vi "OpenAllPods.vi"(11 "Configuration Data":T1) -> (3 "All Pods":T18(array[cluster]))   [LabVIEW 2014]
uses:
  <vilib>/Rock Robotics/WPI/MotorControl/WPI_MotorControlDeviceRef.ctl
  <vilib>/Rock Robotics/WPI/MotorControl/WPI_MotorControlType.ctl
  <vilib>/Rock Robotics/SystemInterfaces/Typedef/FPGA_TypedefDigitalModule.ctl
  <vilib>/Rock Robotics/SystemInterfaces/DIO/FPGA_DIOPWMChannel.ctl
  <vilib>/Rock Robotics/WPI/PWM/WPI_PWMDeadband.ctl
  <vilib>/Rock Robotics/WPI/CAN/Jaguar/SubVIs/WPI_CANJaguar_ControlMode.ctl
  <vilib>/Rock Robotics/WPI/CAN/TalonSRX/WPI_CANTalonSRX_APIControlMode.ctl
  <vilib>/Rock Robotics/WPI/PWM/WPI_PWMTransform_ConPane.ctl
  <vilib>/Rock Robotics/WPI/AnalogChannel/WPI_AnalogChannelDevRef.ctl
  <vilib>/Rock Robotics/SystemInterfaces/Typedef/FPGA_TypedefAnalogModule.ctl
  <vilib>/Rock Robotics/SystemInterfaces/AI/FPGA_AIChannel.ctl
  <vilib>/Rock Robotics/WPI/Encoder/WPI_EncoderDevRef.ctl
  <vilib>/Rock Robotics/SystemInterfaces/Encoder/FPGA_EncoderIdx.ctl
  <vilib>/Rock Robotics/SystemInterfaces/Counter/FPGA_CounterCtrSystemIndex.ctl
  <vilib>/Rock Robotics/WPI/Encoder/WPI_EncoderType.ctl
  <vilib>/Rock Robotics/WPI/MotorControl/WPI_MotorControlOpen Talon.vi
  <vilib>/Rock Robotics/WPI/MotorControl/WPI_MotorControlOpenCANTalonSRX.vi
  <vilib>/Rock Robotics/WPI/Counter/WPI_CounterDigitalInputToDigitalSource.vi
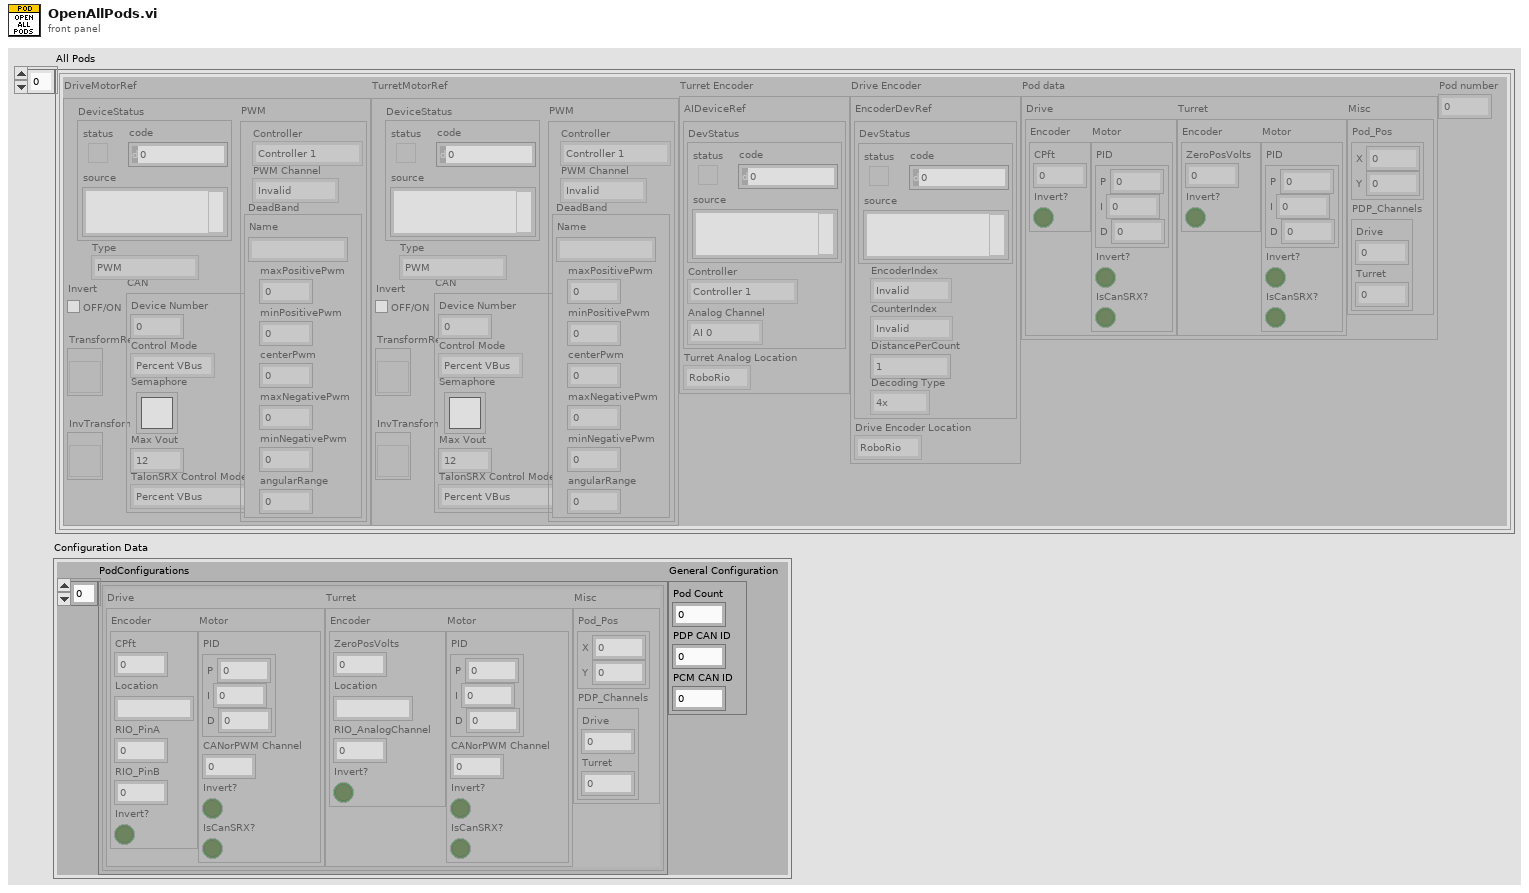
[diagram p1: front panel]
types:
  T1 = cluster{"PodConfigurations":cluster{"Drive":cluster{"Encoder":cluster{"CPft":dbl, "Location":string, "RIO_PinA":i32, "RIO_PinB":i32, "Invert?":bool}, "Motor":cluster{"PID":cluster{"P":dbl, "I":dbl, "D":dbl}, "CANorPWM Channel":i32, "Invert?":bool, "IsCanSRX?":bool}}, "Turret":cluster{"Encoder":cluster{"ZeroPosVolts":dbl, "Location":string, "RIO_AnalogChannel":i32, "Invert?":bool}, "Motor":cluster{"PID":cluster{"P":dbl, "I":dbl, "D":dbl}, "CANorPWM Channel":i32, "Invert?":bool, "IsCanSRX?":bool}}, "Misc":cluster{"Pod_Pos":cluster{"X":dbl, "Y":dbl}, "PDP_Channels":cluster{"Drive":i32, "Turret":i32}}}[], "General Configuration":cluster{"Pod Count":i32, "PDP CAN ID":i32, "PCM CAN ID":i32}}
  T2 = typedef "WPI_MotorControlDeviceRef.ctl" = cluster{"DeviceStatus":errorcluster, "Type":T3, "PWM":cluster{"Controller":T4, "PWM Channel":T5, "DeadBand":T6}, "CAN":cluster{"Device Number":u8, "Control Mode":T7, "Semaphore":T8, "Max Vout":dbl, "TalonSRX Control Mode":T9}, "Invert":bool, "TransformRef":T10, "InvTransformRef":T10}
  T3 = typedef "WPI_MotorControlType.ctl" = enum16{"PWM", "CAN", "CANTalonSRX"}
  T4 = typedef "FPGA_TypedefDigitalModule.ctl" = enum16{"Controller 1"}
  T5 = typedef "FPGA_DIOPWMChannel.ctl" = enum8{"PWM 0", "PWM 1", "PWM 2", "PWM 3", "PWM 4", "PWM 5", "PWM 6", "PWM 7", "PWM 8", "PWM 9", "PWM MXP 0", "PWM MXP 1", "PWM MXP 2", "PWM MXP 3", "PWM MXP 4", "PWM MXP 5", "PWM MXP 6", "PWM MXP 7", "PWM MXP 8", "PWM MXP 9", "Invalid"}
  T6 = typedef "WPI_PWMDeadband.ctl" = cluster{"Name":string, "maxPositivePwm":i32, "minPositivePwm":i32, "centerPwm":i32, "maxNegativePwm":i32, "minNegativePwm":i32, "angularRange":u16}
  T7 = typedef "WPI_CANJaguar_ControlMode.ctl" = enum8{"Percent VBus", "Current", "Speed", "Position", "Voltage"}
  T8 = typedef "Semaphore RefNum" = refnum<k1>
  T9 = typedef "WPI_CANTalonSRX_APIControlMode.ctl" = enum8{"Percent VBus", "Speed", "Position", "Slave", "Unchanged / Invalid"}
  T10 = typedef "WPI_PWMTransform_ConPane.ctl" = refnum<vi>
  T11 = typedef "WPI_AnalogChannelDevRef.ctl" = cluster{"DevStatus":errorcluster, "Controller":T12, "Analog Channel":T13}
  T12 = typedef "FPGA_TypedefAnalogModule.ctl" = enum16{"Controller 1"}
  T13 = typedef "FPGA_AIChannel.ctl" = enum8{"AI 0", "AI 1", "AI 2", "AI 3", "AI MXP 0", "AI MXP 1", "AI MXP 2", "AI MXP 3", "Invalid"}
  T14 = typedef "WPI_EncoderDevRef.ctl" = cluster{"DevStatus":errorcluster, "EncoderIndex":T15, "CounterIndex":T16, "DistancePerCount":dbl, "Decoding Type":T17}
  T15 = typedef "FPGA_EncoderIdx.ctl" = enum8{"Enc 0", "Enc 1", "Enc 2", "Enc 3", "Enc 4", "Enc 5", "Enc 6", "Enc 7", "Invalid"}
  T16 = typedef "FPGA_CounterCtrSystemIndex.ctl" = enum8{"Ctr 0", "Ctr 1", "Ctr 2", "Ctr 3", "Ctr 4", "Ctr 5", "Ctr 6", "Ctr 7", "Invalid"}
  T17 = typedef "WPI_EncoderType.ctl" = enum16{"1x", "2x", "4x"}
  T18 = cluster{"DriveMotorRef":T2, "TurretMotorRef":T2, "Turret Encoder":cluster{"AIDeviceRef":T11, "Turret Analog Location":enum16{"RoboRio", "Drive SRX", "Turret SRX"}}, "Drive Encoder":cluster{"EncoderDevRef":T14, "Drive Encoder Location":enum16{"RoboRio", "Drive SRX", "Turret SRX"}}, "Pod data":cluster{"Drive":cluster{"Encoder":cluster{"CPft":dbl, "Invert?":bool}, "Motor":cluster{"PID":cluster{"P":dbl, "I":dbl, "D":dbl}, "Invert?":bool, "IsCanSRX?":bool}}, "Turret":cluster{"Encoder":cluster{"ZeroPosVolts":dbl, "Invert?":bool}, "Motor":cluster{"PID":cluster{"P":dbl, "I":dbl, "D":dbl}, "Invert?":bool, "IsCanSRX?":bool}}, "Misc":cluster{"Pod_Pos":cluster{"X":dbl, "Y":dbl}, "PDP_Channels":cluster{"Drive":i32, "Turret":i32}}}, "Pod number":i32}[]
  T19 = cluster{"DriveMotorRef":T2, "TurretMotorRef":T2, "Turret Encoder":cluster{"AIDeviceRef":T11, "Turret Analog Location":enum16{"RoboRio", "Drive SRX", "Turret SRX"}}, "Drive Encoder":cluster{"EncoderDevRef":T14, "Drive Encoder Location":enum16{"RoboRio", "Drive SRX", "Turret SRX"}}, "Pod data":cluster{"Drive":cluster{"Encoder":cluster{"CPft":dbl, "Invert?":bool}, "Motor":cluster{"PID":cluster{"P":dbl, "I":dbl, "D":dbl}, "Invert?":bool, "IsCanSRX?":bool}}, "Turret":cluster{"Encoder":cluster{"ZeroPosVolts":dbl, "Invert?":bool}, "Motor":cluster{"PID":cluster{"P":dbl, "I":dbl, "D":dbl}, "Invert?":bool, "IsCanSRX?":bool}}, "Misc":cluster{"Pod_Pos":cluster{"X":dbl, "Y":dbl}, "PDP_Channels":cluster{"Drive":dbl, "Turret":dbl}}}, "Pod number":i32}
  T20 = cluster{"Drive":cluster{"Encoder":cluster{"CPft":dbl, "Location":string, "RIO_PinA":i32, "RIO_PinB":i32, "Invert?":bool}, "Motor":cluster{"PID":cluster{"P":dbl, "I":dbl, "D":dbl}, "CANorPWM Channel":i32, "Invert?":bool, "IsCanSRX?":bool}}, "Turret":cluster{"Encoder":cluster{"ZeroPosVolts":dbl, "Location":string, "RIO_AnalogChannel":i32, "Invert?":bool}, "Motor":cluster{"PID":cluster{"P":dbl, "I":dbl, "D":dbl}, "CANorPWM Channel":i32, "Invert?":bool, "IsCanSRX?":bool}}, "Misc":cluster{"Pod_Pos":cluster{"X":dbl, "Y":dbl}, "PDP_Channels":cluster{"Drive":i32, "Turret":i32}}}[]
  T21 = typedef "WPI_DigitalInputDevRef.ctl" = cluster{"DevStatus":errorcluster, "DIO Channel":T22, "Controller":T4}
  T22 = typedef "FPGA_DIOChannel.ctl" = enum8{"DIO 0", "DIO 1", "DIO 2", "DIO 3", "DIO 4", "DIO 5", "DIO 6", "DIO 7", "DIO 8", "DIO 9", "DIO MXP 0", "DIO MXP 1", "DIO MXP 2", "DIO MXP 3", "DIO MXP 4", "DIO MXP 5", "DIO MXP 6", "DIO MXP 7", "DIO MXP 8", "DIO MXP 9", "DIO MXP 10", "DIO MXP 11", "DIO MXP 12", "DIO MXP 13", "DIO MXP 14", "DIO MXP 15", "Invalid"}
  T23 = typedef "FPGA_CounterEncoderSourceConvertionLVSourceType.ctl" = cluster{"DevStatus":errorcluster, "AnalogTriggerMode?":bool, "DigitalMode":cluster{"Controller":T4, "DIO Channel":T24}, "AnalogTriggerMode":cluster{"AnalogTriggerIndex":T25, "OutputType":T26}}
  T24 = typedef "FPGA_DIODigitalSourceChannel.ctl" = enum8{"DIO 0", "DIO 1", "DIO 2", "DIO 3", "DIO 4", "DIO 5", "DIO 6", "DIO 7", "DIO 8", "DIO 9", "DIO MXP 0", "DIO MXP 1", "DIO MXP 2", "DIO MXP 3", "DIO MXP 4", "DIO MXP 5", "DIO MXP 6", "DIO MXP 7", "DIO MXP 8", "DIO MXP 9", "DIO MXP 10", "DIO MXP 11", "DIO MXP 12", "DIO MXP 13", "DIO MXP 14", "DIO MXP 15", "Disabled"}
  T25 = typedef "FPGA_AnalogTriggerIndex.ctl" = enum8{"Trig 0", "Trig 1", "Trig 2", "Trig 3", "Trig 4", "Trig 5", "Trig 6", "Trig 7", "Invalid"}
  T26 = typedef "FPGA_AnalogTriggerOutType.ctl" = enum16{"InWindow", "TriggerState", "Rising", "Falling"}
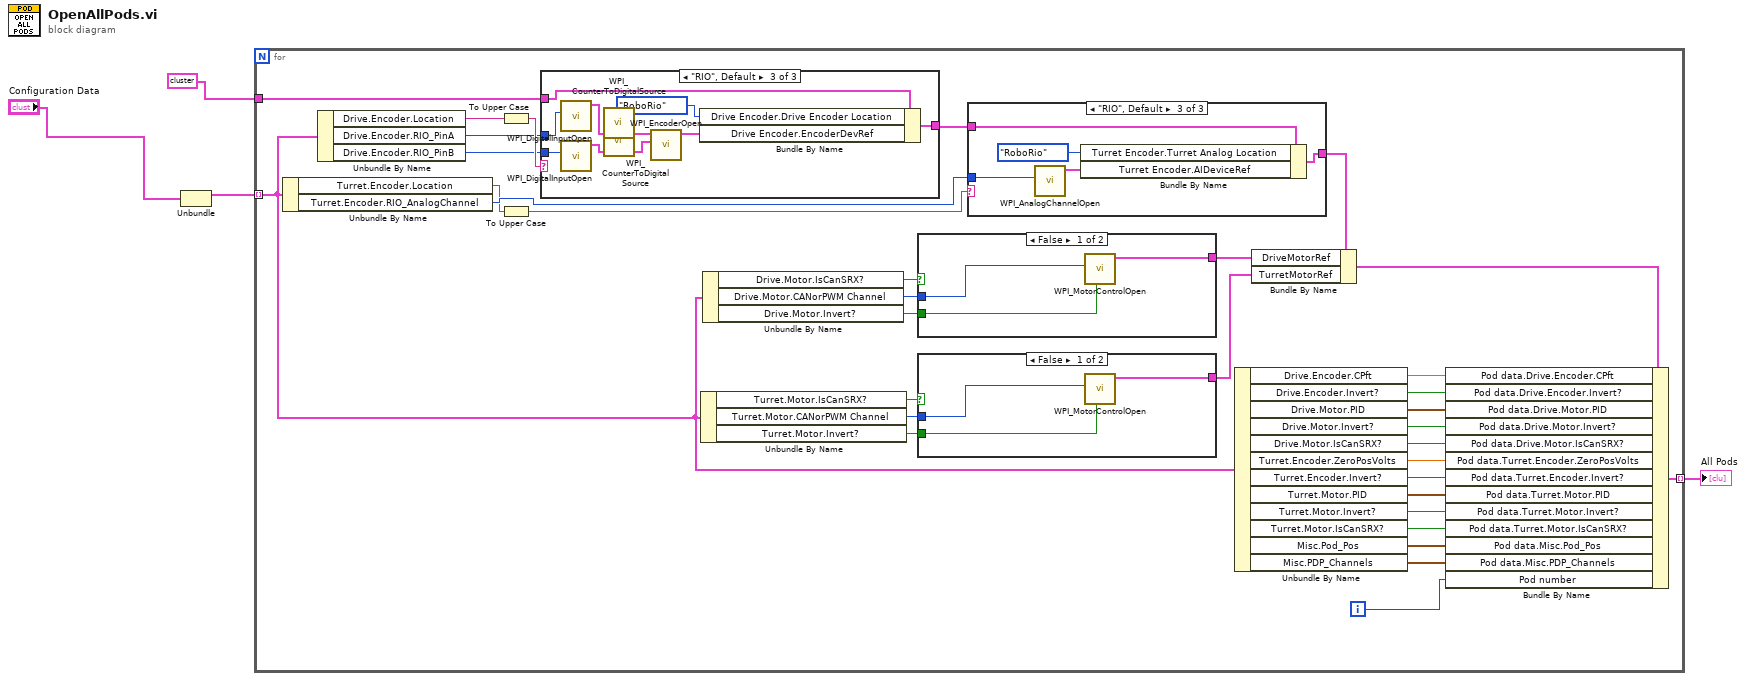
[diagram p0: block diagram]
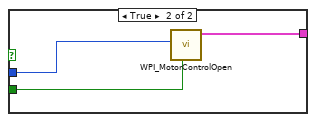
[diagram p2: hidden frame]
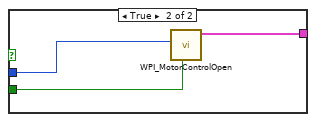
[diagram p3: hidden frame]
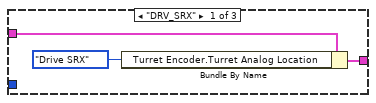
[diagram p4: hidden frame]
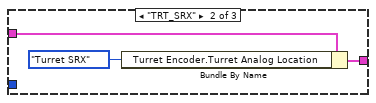
[diagram p5: hidden frame]
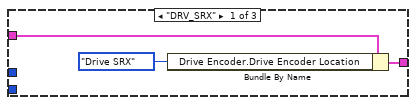
[diagram p6: hidden frame]
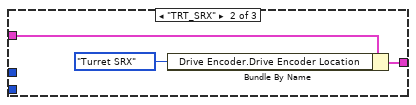
[diagram p7: hidden frame]
diagram:
  n1 = Unbundle("Configuration Data") -> ("PodConfigurations"=w4:T20)  [unwired: 1 out]
  n2 = for {
    tunnel: w4 -> [w18] mode=indexing
    tunnel: T19 {"DriveMotorRef"={"DeviceStatus"={"status"=FALSE, "code"=0, "source"=""}, "Type"=enum."PWM", "PWM"={"Controller"=enum."Controller 1", "PWM Channel"=enum."Invalid", "DeadBand"={"Name"="", "maxPositivePwm"=0, "minPositivePwm"=0, "centerPwm"=0, "maxNegativePwm"=0, "minNegativePwm"=0, "angularRange"=0}}, "CAN"={"Device Number"=0, "Control Mode"=enum."Percent VBus", "Semaphore"=refnum, "Max Vout"=12.0, "TalonSRX Control Mode"=enum."Percent VBus"}, "Invert"=FALSE, "TransformRef"=refnum, "InvTransformRef"=refnum}, "TurretMotorRef"={"DeviceStatus"={"status"=FALSE, "code"=0, "source"=""}, "Type"=enum."PWM", "PWM"={"Controller"=enum."Controller 1", "PWM Channel"=enum."Invalid", "DeadBand"={"Name"="", "maxPositivePwm"=0, "minPositivePwm"=0, "centerPwm"=0, "maxNegativePwm"=0, "minNegativePwm"=0, "angularRange"=0}}, "CAN"={"Device Number"=0, "Control Mode"=enum."Percent VBus", "Semaphore"=refnum, "Max Vout"=12.0, "TalonSRX Control Mode"=enum."Percent VBus"}, "Invert"=FALSE, "TransformRef"=refnum, "InvTransformRef"=refnum}, "Turret Encoder"={"AIDeviceRef"={"DevStatus"={"status"=FALSE, "code"=0, "source"=""}, "Controller"=enum."Controller 1", "Analog Channel"=enum."AI 0"}, "Turret Analog Location"=enum."RoboRio"}, "Drive Encoder"={"EncoderDevRef"={"DevStatus"={"status"=FALSE, "code"=0, "source"=""}, "EncoderIndex"=enum."Invalid", "CounterIndex"=enum."Invalid", "DistancePerCount"=1.0, "Decoding Type"=enum."4x"}, "Drive Encoder Location"=enum."RoboRio"}, "Pod data"={"Drive"={"Encoder"={"CPft"=0.0, "Invert?"=FALSE}, "Motor"={"PID"={"P"=0.0, "I"=0.0, "D"=0.0}, "Invert?"=FALSE, "IsCanSRX?"=FALSE}}, "Turret"={"Encoder"={"ZeroPosVolts"=0.0, "Invert?"=FALSE}, "Motor"={"PID"={"P"=0.0, "I"=0.0, "D"=0.0}, "Invert?"=FALSE, "IsCanSRX?"=FALSE}}, "Misc"={"Pod_Pos"={"X"=0.0, "Y"=0.0}, "PDP_Channels"={"Drive"=0.0, "Turret"=0.0}}}, "Pod number"=0} ("Pod") -> [w36]
    tunnel: [w19] -> w2 mode=indexing
    i -> [w5]
    n3 = Unbundle By Name(w18) -> ("Turret.Encoder.Location"=w31:string, "Turret.Encoder.RIO_AnalogChannel"=w33:i32)
    n4 = Unbundle By Name(w18) -> ("Drive.Encoder.Location"=w38:string, "Drive.Encoder.RIO_PinA"=w35:i32, "Drive.Encoder.RIO_PinB"=w34:i32)
    n5 = To Upper Case(1:w38) -> (0:w37:string)
    n6 = To Upper Case(1:w31) -> (0:w32:string)
    n7 = case shown="\"RIO\", Default" w37 {
      tunnel: w36 -> [w63 w67 w76]
      tunnel: [w62 w66 w75] -> w30
      tunnel: w35 -> [_ _ w69]
      tunnel: w34 -> [_ _ w68]
      frame "DRV_SRX" {
        n8 = Bundle By Name(cluster=w63, "Drive Encoder.Drive Encoder Location"=enum16{"RoboRio", "Drive SRX", "Turret SRX"}."Drive SRX") -> (w62:T19)
      }
      frame "TRT_SRX" {
        n9 = Bundle By Name(cluster=w67, "Drive Encoder.Drive Encoder Location"=enum16{"RoboRio", "Drive SRX", "Turret SRX"}."Turret SRX") -> (w66:T19)
      }
      frame "RIO", Default {
        n10 = call <vilib>:"WPI_DigitalInputOpen.vi"("DIO Channel"=w69) -> ("DigitalInputDevRef"=w72:T21)  [unwired: 2 in, 8 out]
        n11 = call <vilib>:"WPI_DigitalInputOpen.vi"("DIO Channel"=w68) -> ("DigitalInputDevRef"=w73:T21)  [unwired: 2 in, 8 out]
        n12 = call-poly <vilib>:"WPI_CounterToDigitalSource.vi"("DigitalInputDevRef"=w72) -> ("Digital Source"=w71:T23)  [unwired: 6 out]
        n13 = call-poly <vilib>:"WPI_CounterToDigitalSource.vi"("DigitalInputDevRef"=w73) -> ("Digital Source"=w74:T23)  [unwired: 6 out]
        n14 = call <vilib>:"WPI_EncoderOpen.vi"("BSource"=w74, "ASource"=w71) -> ("EncoderDevRef"=w70:T14)  [unwired: 6 in, 3 out]
        n15 = Bundle By Name(cluster=w76, "Drive Encoder.Drive Encoder Location"=enum16{"RoboRio", "Drive SRX", "Turret SRX"}."RoboRio", "Drive Encoder.EncoderDevRef"=w70) -> (w75:T19)
      }
    }
    n16 = Unbundle By Name(w18) -> ("Turret.Motor.IsCanSRX?"=w22:bool, "Turret.Motor.CANorPWM Channel"=w23:i32, "Turret.Motor.Invert?"=w24:bool)
    n17 = Unbundle By Name(w18) -> ("Drive.Motor.IsCanSRX?"=w29:bool, "Drive.Motor.CANorPWM Channel"=w28:i32, "Drive.Motor.Invert?"=w27:bool)
    n18 = case shown="False" w29 {
      tunnel: w28 -> [w47 w50]
      tunnel: w27 -> [w46 w49]
      tunnel: [w45 w48] -> w25
      frame False {
        n19 = call-poly <vilib>:"WPI_MotorControlOpen.vi"("Invert"=w46, "PWM Channel"=w47) -> ("MotorControlDeviceRef"=w45:T2)  [unwired: 8 in, 1 out]
      }
      frame True {
        n20 = call-poly <vilib>:"WPI_MotorControlOpen.vi"("Invert"=w49, "Device Number"=w50) -> ("MotorControlDeviceRef"=w48:T2)  [unwired: 8 in, 1 out]
      }
    }
    n21 = case shown="False" w22 {
      tunnel: w23 -> [w41 w44]
      tunnel: w24 -> [w40 w43]
      tunnel: [w39 w42] -> w21
      frame False {
        n22 = call-poly <vilib>:"WPI_MotorControlOpen.vi"("Invert"=w40, "PWM Channel"=w41) -> ("MotorControlDeviceRef"=w39:T2)  [unwired: 8 in, 1 out]
      }
      frame True {
        n23 = call-poly <vilib>:"WPI_MotorControlOpen.vi"("Invert"=w43, "Device Number"=w44) -> ("MotorControlDeviceRef"=w42:T2)  [unwired: 8 in, 1 out]
      }
    }
    n24 = case shown="\"RIO\", Default" w32 {
      tunnel: w30 -> [w52 w56 w60]
      tunnel: [w51 w55 w59] -> w26
      tunnel: w33 -> [_ _ w58]
      frame "DRV_SRX" {
        n25 = Bundle By Name(cluster=w52, "Turret Encoder.Turret Analog Location"=enum16{"RoboRio", "Drive SRX", "Turret SRX"}."Drive SRX" ("Drive Encoder.Drive Encoder Location")) -> (w51:T19)
      }
      frame "TRT_SRX" {
        n26 = Bundle By Name(cluster=w56, "Turret Encoder.Turret Analog Location"=enum16{"RoboRio", "Drive SRX", "Turret SRX"}."Turret SRX" ("Drive Encoder.Drive Encoder Location")) -> (w55:T19)
      }
      frame "RIO", Default {
        n27 = call <vilib>:"WPI_AnalogChannelOpen.vi"("Analog Channel"=w58) -> ("AIDeviceRef"=w57:T11)  [unwired: 9 in, 1 out]
        n28 = Bundle By Name(cluster=w60, "Turret Encoder.Turret Analog Location"=enum16{"RoboRio", "Drive SRX", "Turret SRX"}."RoboRio" ("Drive Encoder.Drive Encoder Location"), "Turret Encoder.AIDeviceRef"=w57) -> (w59:T19)
      }
    }
    n29 = Unbundle By Name(w18) -> ("Drive.Encoder.CPft"=w17:dbl, "Drive.Encoder.Invert?"=w16:bool, "Drive.Motor.PID"=w15:cluster{"P":dbl, "I":dbl, "D":dbl}, "Drive.Motor.Invert?"=w14:bool, "Drive.Motor.IsCanSRX?"=w13:bool, "Turret.Encoder.ZeroPosVolts"=w12:dbl, "Turret.Encoder.Invert?"=w11:bool, "Turret.Motor.PID"=w10:cluster{"P":dbl, "I":dbl, "D":dbl}, "Turret.Motor.Invert?"=w9:bool, "Turret.Motor.IsCanSRX?"=w7:bool, "Misc.Pod_Pos"=w8:cluster{"X":dbl, "Y":dbl}, "Misc.PDP_Channels"=w6:cluster{"Drive":i32, "Turret":i32})
    n30 = Bundle By Name(cluster=w26, "DriveMotorRef"=w25, "TurretMotorRef"=w21) -> (w20:T19)
    n31 = Bundle By Name(cluster=w20, "Pod data.Drive.Encoder.CPft"=w17, "Pod data.Drive.Encoder.Invert?"=w16, "Pod data.Drive.Motor.PID"=w15, "Pod data.Drive.Motor.Invert?"=w14, "Pod data.Drive.Motor.IsCanSRX?"=w13, "Pod data.Turret.Encoder.ZeroPosVolts"=w12, "Pod data.Turret.Encoder.Invert?"=w11, "Pod data.Turret.Motor.PID"=w10, "Pod data.Turret.Motor.Invert?"=w9, "Pod data.Turret.Motor.IsCanSRX?"=w7, "Pod data.Misc.Pod_Pos"=w8, "Pod data.Misc.PDP_Channels"=w6, "Pod number"=w5) -> (w19:T19)
  }
  "All Pods" <- w2
